vi "Set_Control_Values_by_Index_(Sgnl).vi"(7 "Control References":refnum<vi>[](array[refnum]), 8 "error in (no error)":errorcluster, 9 "appended array":variant[](array[variant]), 11 "VI Refnum":refnum<vi>) -> (0 "error out":errorcluster)   [LabVIEW 2015]
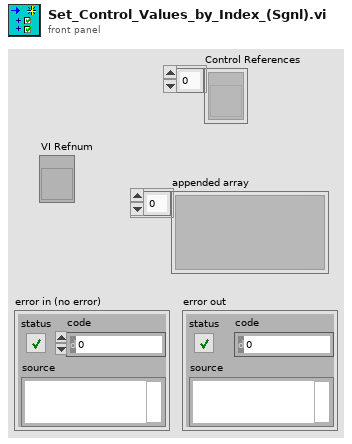
[diagram p1: front panel]
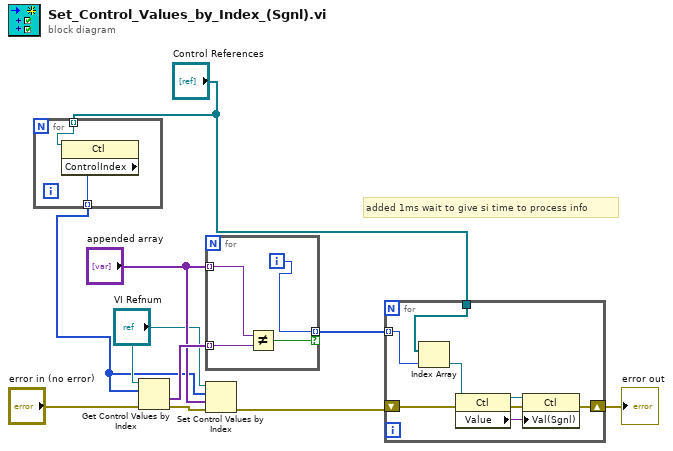
[diagram p0: block diagram]
diagram:
  # "added 1ms wait to give si time to process info"
  n1 = for {
    tunnel: "Control References" -> [w12] mode=indexing
    tunnel: [w11] -> w1 mode=indexing
    n2 = property class="Ctl"(reference=w12) -> ("ControlIndex"=w11:i32)  [unwired: 1 in, 2 out]
  }
  n3 = Get Control Values by Index(0:"VI Refnum", 1:w1, 3:"error in (no error)") -> (10:w10:variant[], 11:w8:errorcluster)
  n4 = for {
    tunnel: "appended array" -> [w16] mode=indexing
    tunnel: w10 -> [w15] mode=indexing
    tunnel: [w13] -> w7 mode=indexing if=w14
    i -> [w13]
    n5 = Not Equal?(x=w16, y=w15) -> (x != y?=w14:bool)
  }
  n6 = Set Control Values by Index(0:"VI Refnum", 1:w1, 2:"appended array", 3:w8) -> (11:w4:errorcluster)
  n7 = for {
    tunnel: w7 -> [w18] mode=indexing
    shift-right: [w24] -> w5
    shift-left: w4 -> [w23]
    tunnel: "Control References" -> [w19]
    n8 = Index Array(array=w19, index=w18) -> (element=w17:refnum<vi>)
    n9 = property class="Ctl"(reference=w17, error in=w23) -> (reference out=w21:refnum<vi>, error out=w22:errorcluster, "Value"=w20:variant)
    n10 = property class="Ctl"(reference=w21, error in=w22, "Val(Sgnl)"=w20) -> (error out=w24:errorcluster)  [unwired: 1 out]
  }
  "error out" <- w5
